vi "数字量输出自动检测.vi"(11 "测试值":enum16{"0", "1"}(ring)) -> (2 "测试结果":string)   [LabVIEW 2010]
uses:
  全局量/全局_配置.vi
panel:
  in  "CAN端口":u16
  out "结束？":bool
  in  "同步_2":i32
  in  "同步_1":i32
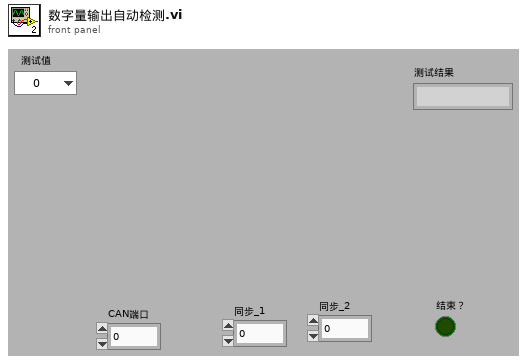
[diagram p1: front panel]
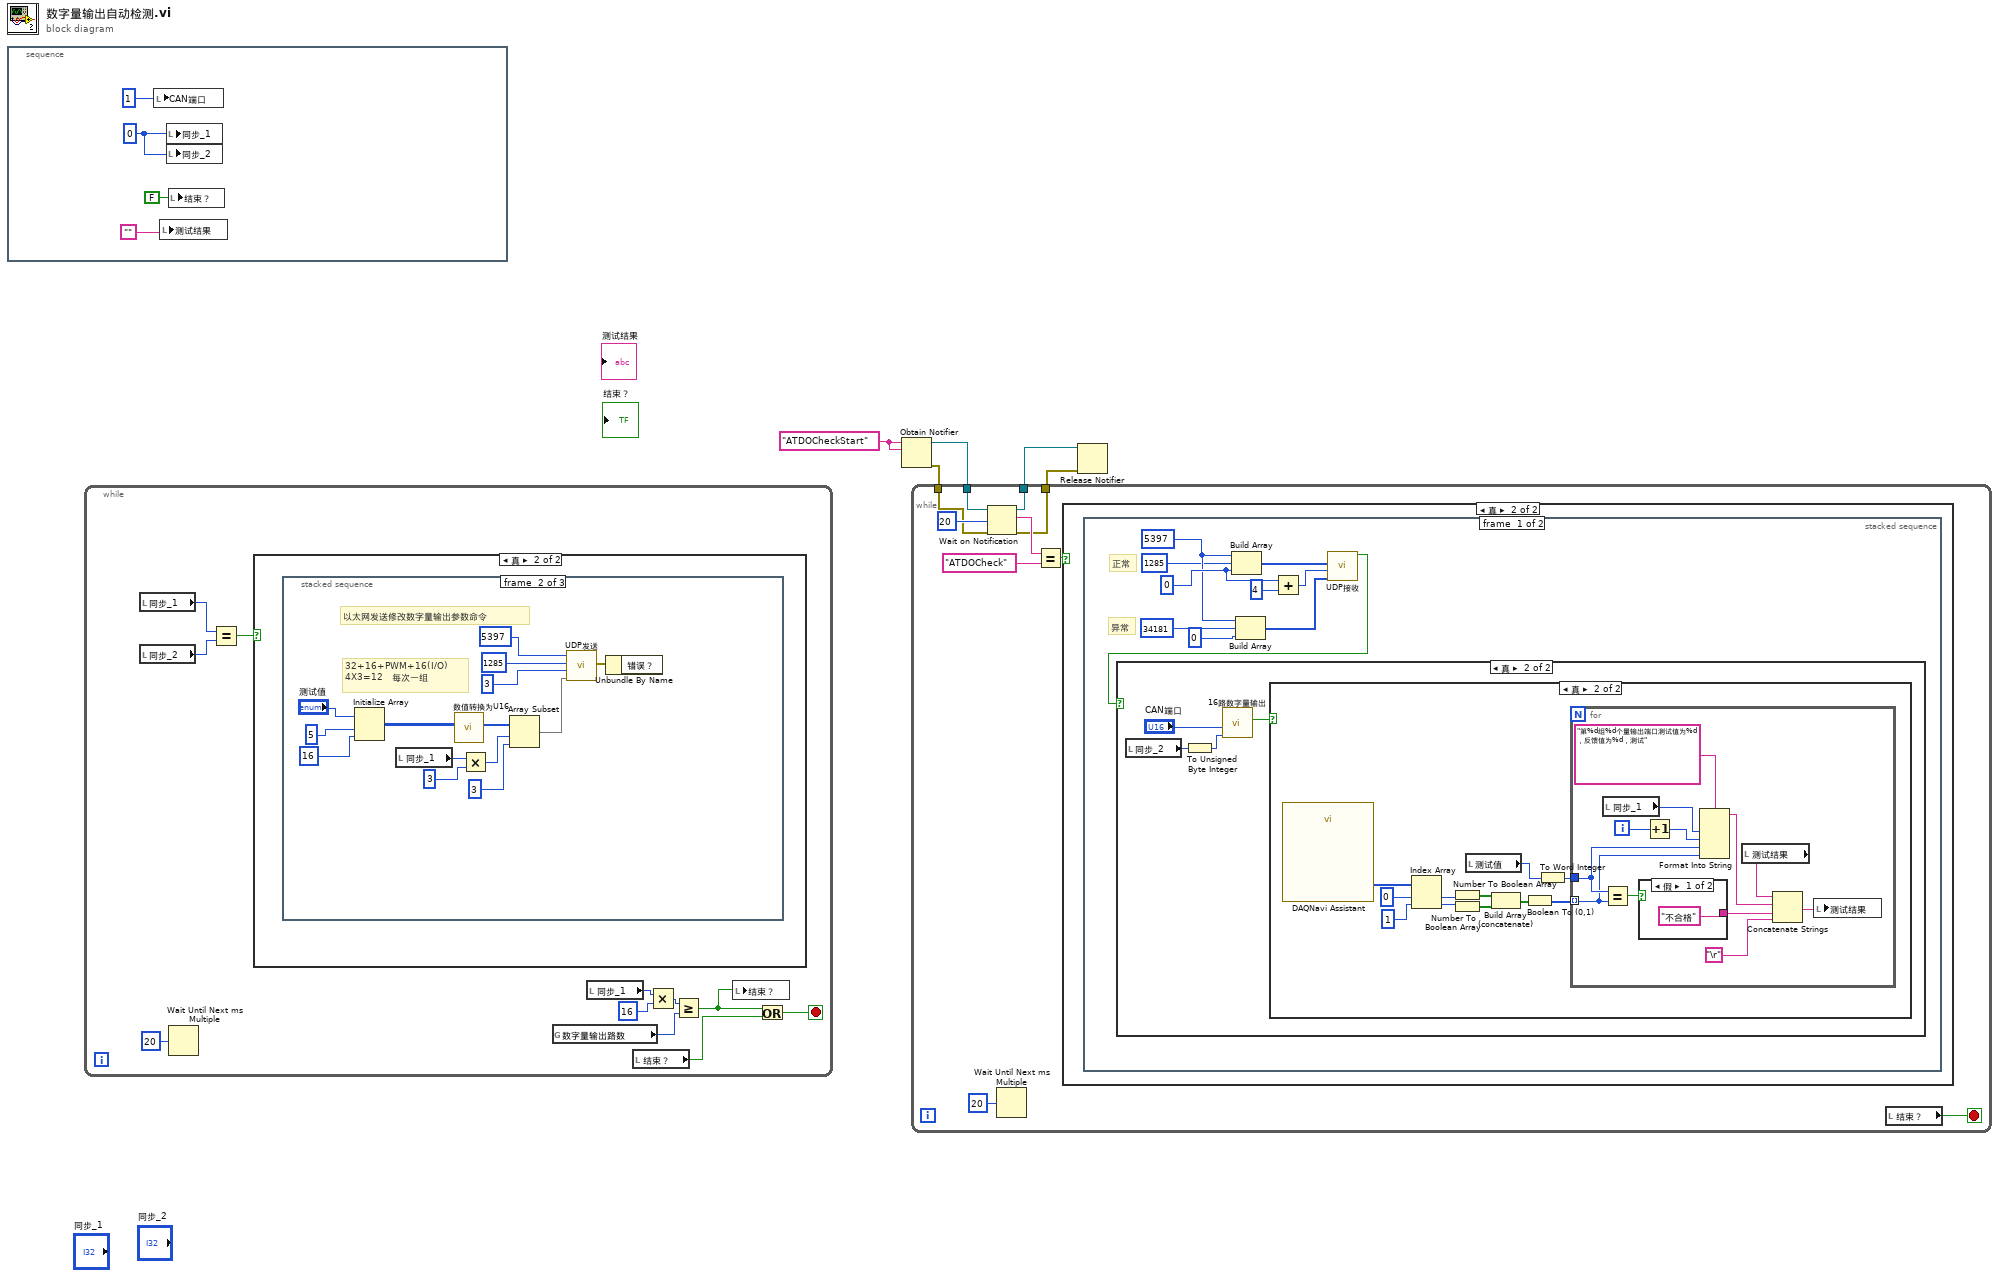
[diagram p0: block diagram]
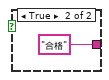
[diagram p5: hidden frame]
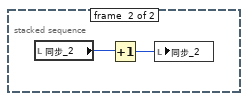
[diagram p6: hidden frame]
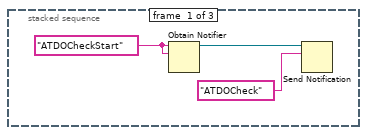
[diagram p8: hidden frame]
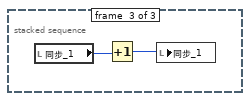
[diagram p9: hidden frame]
diagram:
  w5 = "ATDOCheckStart" ("名称（未命名）")
  n1 = stacked-sequence {
    frame #0 {
      w9 = 0 ("同步_1")
      n2 = local write "CAN端口"(u16 1 ("CAN端口")) -> ()
      n3 = local write "测试结果"("") -> ()
      n4 = local write "同步_1"(w9) -> ()
      n5 = local write "同步_2"(w9) -> ()
      n6 = local write "结束？"(FALSE ("结束？")) -> ()
    }
  }
  n7 = while {
    stop <- w12 stop-if-true
    n8 = local read "同步_1"() -> (w20:i32)
    n9 = local read "同步_2"() -> (w19:i32)
    n10 = Wait Until Next ms Multiple(millisecond multiple=u32 20 ("毫秒倍数")) -> ()  [unwired: 1 out]
    n11 = Equal?(x=w20, y=w19) -> (x = y?=w18:bool)
    n12 = case shown="真" w18 {
      frame False {
      }
      frame True {
        n13 = stacked-sequence {
          frame #0 {
            w22 = "ATDOCheckStart" ("名称（未命名）")
            n14 = Obtain Notifier(name (unnamed)=w22, notification data type=w22) -> (notifier out=w21:refnum<notifier>)  [unwired: 2 in, 2 out]
            n15 = Send Notification(notification="ATDOCheck" ("通知"), notifier=w21) -> ()  [unwired: 1 in, 2 out]
          }
          frame #1 {
            # "32+16+PWM+16(I/O)\n4X3=12   每次一组"
            # "以太网发送修改数字量输出参数命令"
            n16 = Initialize Array("测试值", 5 ("维数大小"), 16 ("维数大小")) -> (w29:enum16{"0", "1"}[][])
            n17 = local read "同步_1"() -> (w32:i32)
            n18 = call "数值转换为U16.vi"("数值数组输入"=w29) -> ("U16输出"=w27:u16[])  [unwired: 10 in]
            n19 = Multiply(x=w32, y=3 ("长度")) -> (x*y=w26:i32)
            n20 = Array Subset(array=w27, index=w26, length=3 ("长度")) -> (w24:u16[])
            n21 = call "UDP发送.vi"("发送数据"=w24, "数据区字长"=u16 3, "报文类型"=u16 1285, "发送方标识"=u16 5397) -> ("Error"=w37:cluster{"错误？":bool, "数值":i32, "字符串":string})  [unwired: 6 in]
            n22 = Unbundle By Name(w37) -> ()  [unwired: 1 out]
          }
          frame #2 {
            n23 = local read "同步_1"() -> (w39:i32)
            n24 = Increment(x=w39) -> (x+1=w38:i32)
            n25 = local write "同步_1"(w38) -> ()
          }
        }
      }
    }
    n26 = global read "全局_配置.vi" "数字量输出路数"() -> (w13:i32)
    n27 = local read "同步_1"() -> (w16:i32)
    n28 = local read "结束？"() -> (w11:bool)
    n29 = Multiply(x=w16, y=16) -> (x*y=w14:i32)
    n30 = Greater Or Equal?(x=w14, y=w13) -> (x >= y?=w10:bool)
    n31 = local write "结束？"(w10) -> ()
    n32 = Or(x=w10, y=w11) -> (x .or. y?=w12:bool)
  }
  n33 = Obtain Notifier(name (unnamed)=w5, notification data type=w5) -> (notifier out=w4:refnum<notifier>, error out=w3:errorcluster)  [unwired: 2 in, 1 out]
  n34 = while {
    tunnel: w4 -> [w49]
    tunnel: w3 -> [w45]
    tunnel: [w44] -> w2
    tunnel: [w43] -> w1
    stop <- w41 stop-if-true
    n35 = Wait on Notification(notifier=w49, timeout in ms (-1)=20 ("超时毫秒(-1)"), error in (no error)=w45) -> (notifier out=w44:refnum<notifier>, notification=w47:string, error out=w43:errorcluster)  [unwired: 1 in, 1 out]
    n36 = Wait Until Next ms Multiple(millisecond multiple=u32 20 ("毫秒倍数")) -> ()  [unwired: 1 out]
    n37 = Equal?(x=w47, y="ATDOCheck" ("通知")) -> (x = y?=w42:bool)
    n38 = case shown="真" w42 {
      frame False {
      }
      frame True {
        n39 = stacked-sequence {
          frame #0 {
            w57 = u16 0
            w54 = u16 5397
            # "异常"
            # "正常"
            n40 = Build Array(w54, u16 1285, w57) -> (w52:u16[])
            n41 = Build Array(w54, u16 34181, u16 0 ("元素")) -> (w55:u16[])
            n42 = Add(x=w57, y=u16 4) -> (x+y=w59:u16)
            n43 = call "UDP接收.vi"("匹配帧信息_异常"=w55, "长度"=w59, "匹配帧信息_正常"=w52) -> ("正常_找到?"=w50:bool)  [unwired: 5 in, 3 out]
            n44 = case shown="真" w50 {
              frame False {
              }
              frame True {
                n45 = local read "同步_2"() -> (w61:i32)
                n46 = To Unsigned Byte Integer(number=w61) -> (unsigned 8bit integer=w62:u8)
                n47 = call "16路数字量输出.vi"("第几组数据"=w62, "CAN端口"="CAN端口") -> ("成功?"=w60:bool)  [unwired: 9 in]
                n48 = case shown="真" w60 {
                  frame False {
                  }
                  frame True {
                    n49 = call "DAQNavi Assistant"() -> ("dataOut(U8Array)"=w67:u8[])  [unwired: 2 in, 17 out]
                    n50 = Index Array(array=w67, index #1=0 ("索引"), index #2=1 ("索引")) -> (element #1=w70:u8, element #2=w71:u8)
                    n51 = Number To Boolean Array(number=w70) -> (Boolean array=w73:bool[])
                    n52 = Number To Boolean Array(number=w71) -> (Boolean array=w74:bool[])
                    n53 = local read "测试值"() -> (w64:enum16{"0", "1"})
                    n54 = Build Array (concatenate)(w73, w74) -> (w72:bool[])
                    n55 = Boolean To (0,1)(Boolean=w72) -> (0, 1=w66:i16[])
                    n56 = To Word Integer(number=w64) -> (16bit integer=w65:i16)
                    n57 = for {
                      tunnel: w66 -> [w75] mode=indexing
                      tunnel: w65 -> [w76]
                      i -> [w83]
                      n58 = local read "同步_1"() -> (w84:i32)
                      n59 = Equal?(x=w76, y=w75) -> (x = y?=w86:bool)
                      n60 = case shown="假" w86 {
                        tunnel: ["不合格" "合格"] -> w80
                        frame False {
                        }
                        frame True {
                        }
                      }
                      n61 = Increment(x=w83) -> (x+1=w82:i32)
                      n62 = Format Into String(format string="第%d组%d个量输出端口测试值为%d，反馈值为%d，测试", w84, w82, w76, w75) -> (resulting string=w81:string)  [unwired: 2 in, 1 out]
                      n63 = local read "测试结果"() -> (w78:string)
                      n64 = Concatenate Strings(w78, w81, w80, "\r") -> (w77:string)
                      n65 = local write "测试结果"(w77) -> ()
                    }
                  }
                }
              }
            }
          }
          frame #1 {
            n66 = local read "同步_2"() -> (w90:i32)
            n67 = Increment(x=w90) -> (x+1=w89:i32)
            n68 = local write "同步_2"(w89) -> ()
          }
        }
      }
    }
    n69 = local read "结束？"() -> (w41:bool)
  }
  n70 = Release Notifier(notifier=w2, error in (no error)=w1) -> ()  [unwired: 1 in, 3 out]
